vi "EnFlo_Tun_Heater_Control.vi"(1 "Ch Names":string[](array[string]), 2 "Values":dbl[](array[numeric]) format="%.2f") -> ()   [LabVIEW 2010]
uses:
  ADAM_Global.vi
  <vilib>/Analysis/NI_AALPro.lvlib
  <vilib>/Analysis/NI_AALBase.lvlib
panel:
  in  "Total History":i32=80
  out "Proportional Term":dbl format="%#.1f"
  out "Control Sum":dbl format="%#.1f"
  out "Differential Term":dbl format="%#.1f"
  in  "Derivative History":i32=25
  out "Integral Term":dbl format="%#.1f"
  in  "Kp":dbl=6.0 format="%.2f"
  in  "Kd":dbl=150.0 format="%.2f"
  in  "Ki":dbl=0.05 format="%.2f"
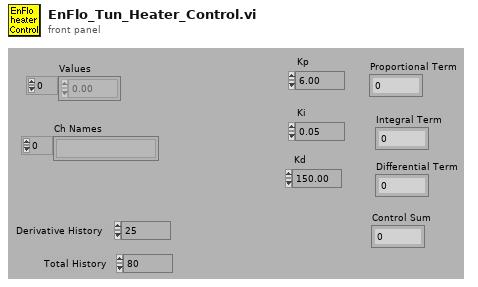
[diagram p1: front panel]
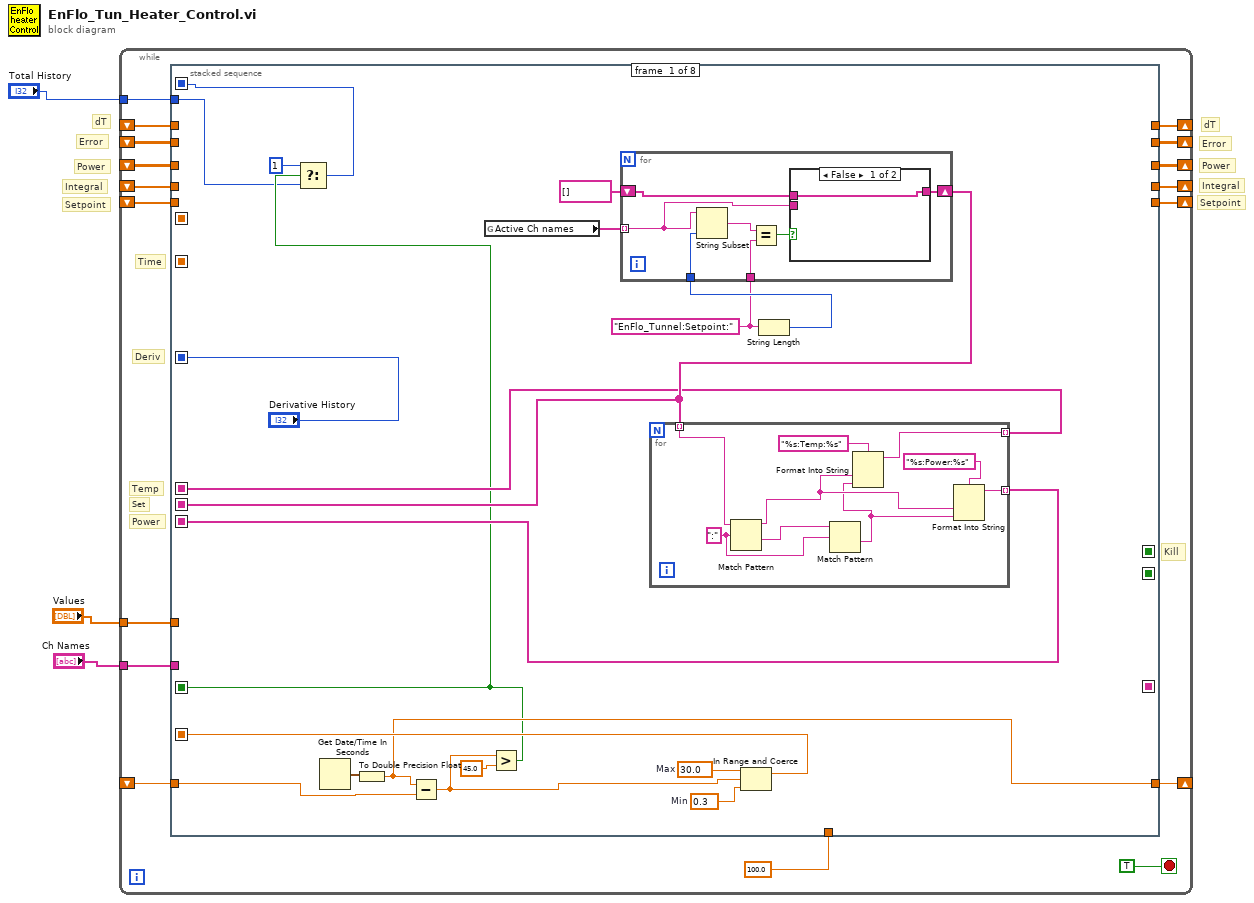
[diagram p0: block diagram]
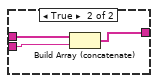
[diagram p2: hidden frame]
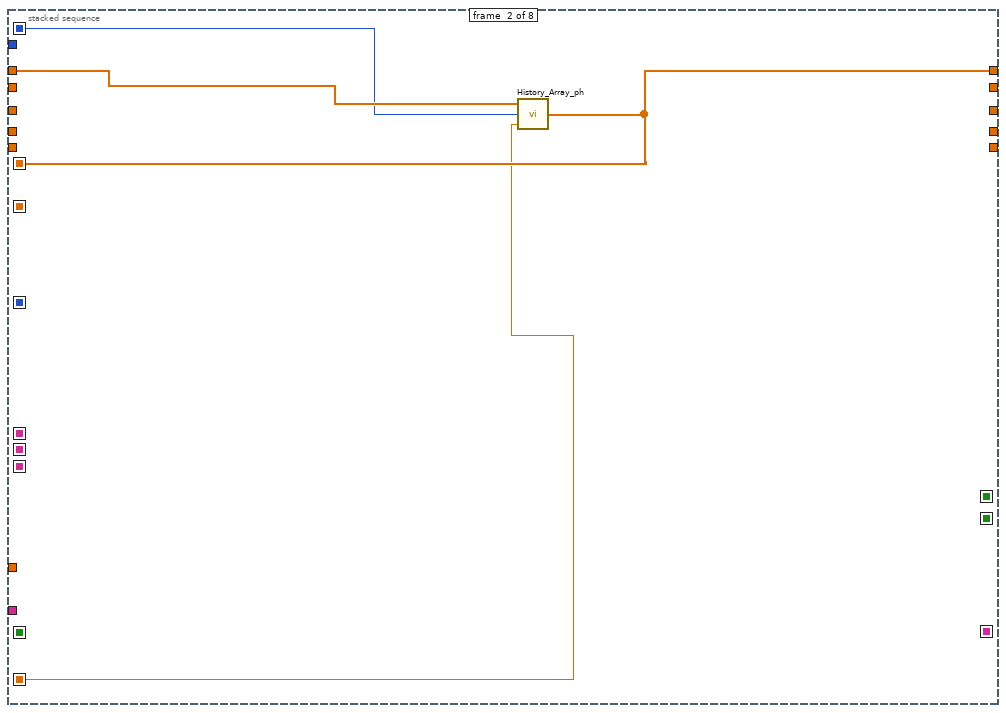
[diagram p3: hidden frame]
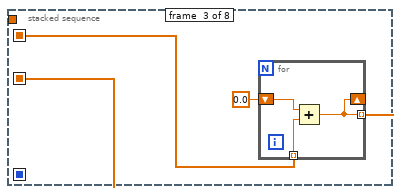
[diagram p4: hidden frame]
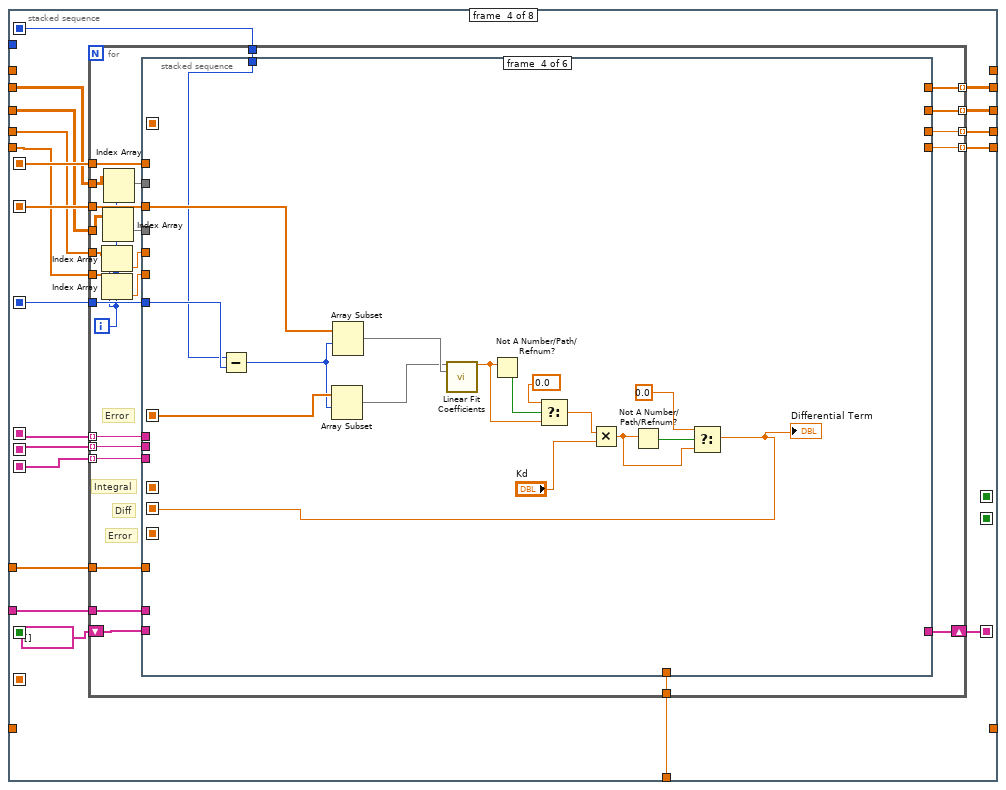
[diagram p5: hidden frame]
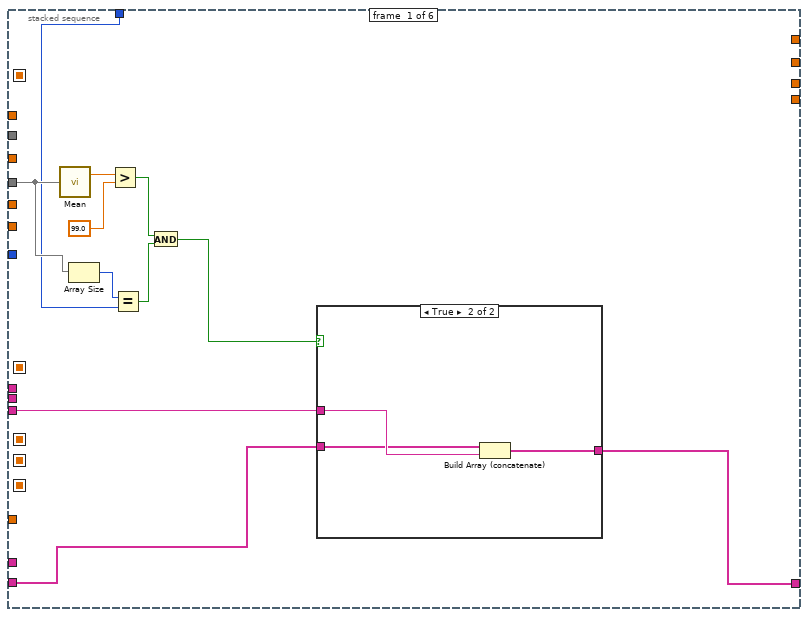
[diagram p6: hidden frame]
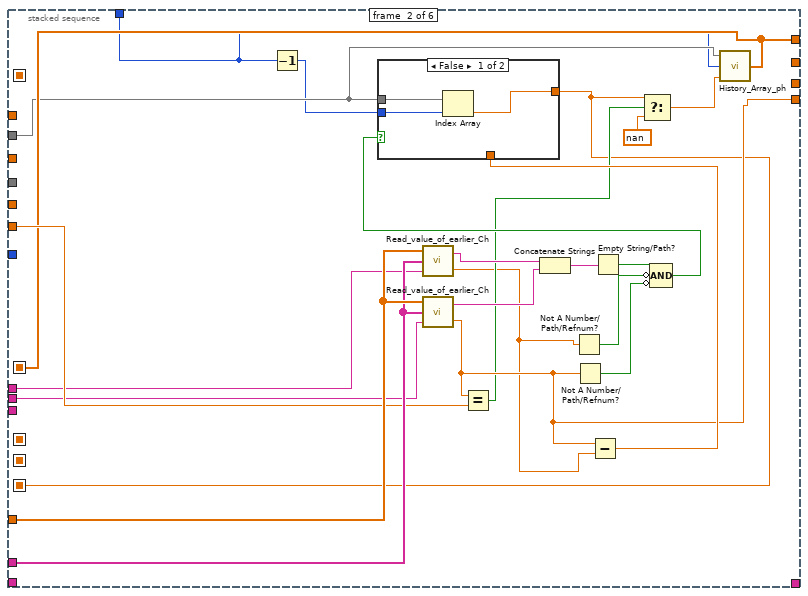
[diagram p8: hidden frame]
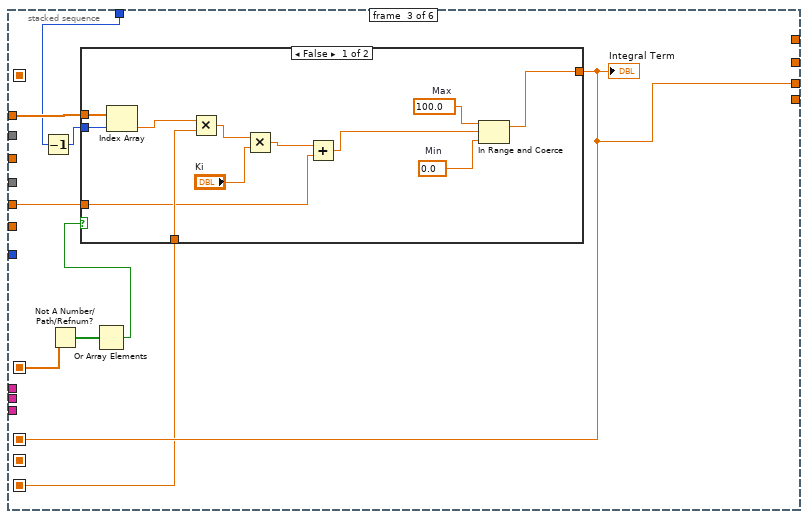
[diagram p10: hidden frame]
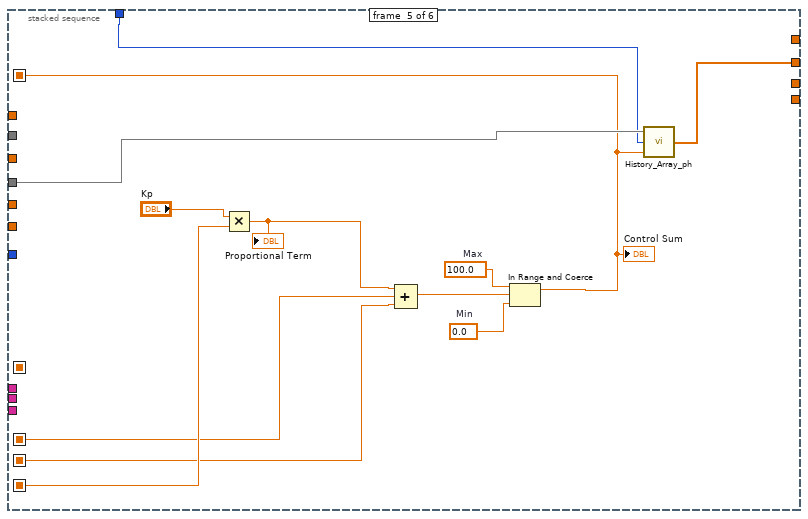
[diagram p12: hidden frame]
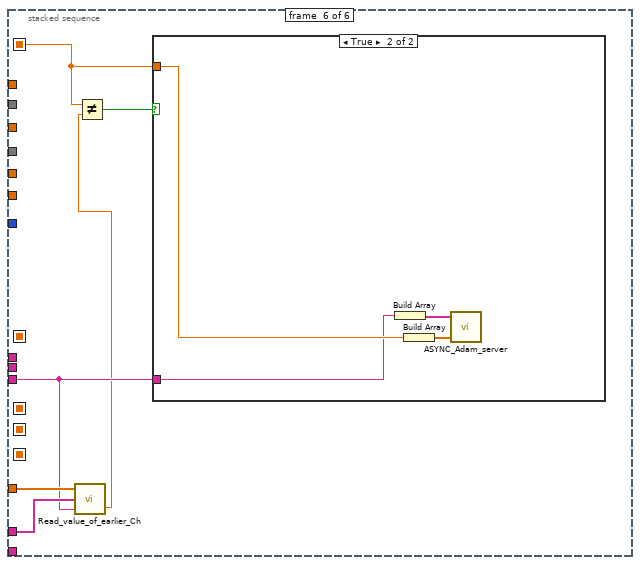
[diagram p13: hidden frame]
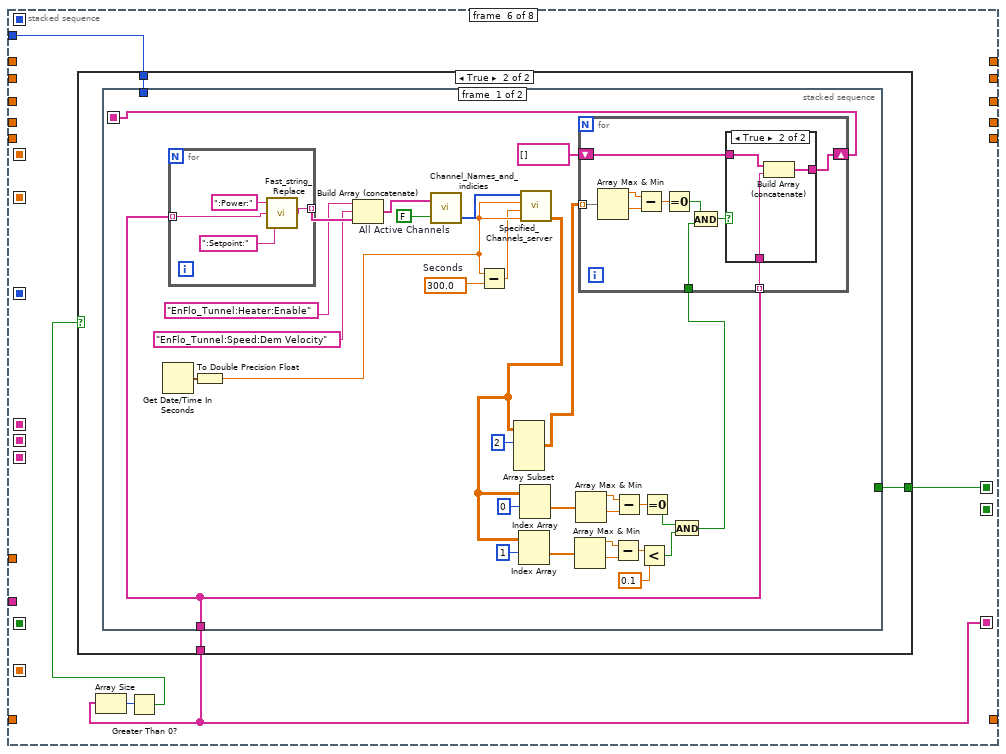
[diagram p16: hidden frame]
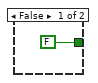
[diagram p17: hidden frame]
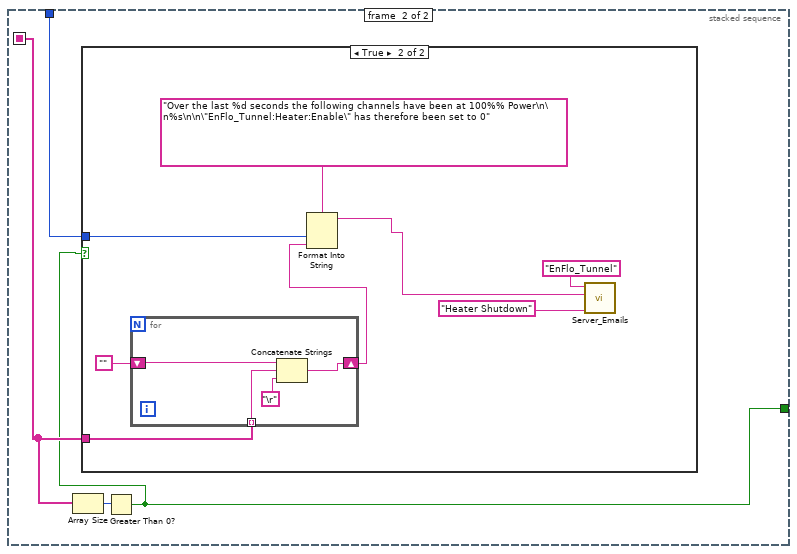
[diagram p19: hidden frame]
diagram:
  # "Setpoint"
  # "Integral"
  # "Power"
  # "Error"
  # "dT"
  # "Setpoint"
  # "Power"
  # "Integral"
  # "Error"
  # "dT"
  n1 = while {
    shift-right: [w18] -> _
    shift-left: _ -> [w19]
    shift-right: [w14] -> _
    shift-left: _ -> [w17]
    shift-right: [w16] -> _
    shift-left: _ -> [w15]
    shift-right: [w12] -> _
    shift-left: _ -> [w13]
    shift-right: [w10] -> _
    shift-left: _ -> [w11]
    shift-right: [w8] -> _
    shift-left: _ -> [w9]
    tunnel: "Total History" -> [w7]
    tunnel: "Ch Names" -> [w5]
    tunnel: "Values" -> [w4]
    stop <- TRUE stop-if-true
    # "Kill"
    # "Power"
    # "Set"
    # "Temp"
    # "Deriv"
    # "Time"
    n2 = stacked-sequence {
      seq-local: [_ w64 _ _ _ _ _ _] -> [_ _ w66 w89 _ _ _ _]
      seq-local: [_ _ w65 _ _ _ _ _] -> [_ _ _ w88 _ _ _ _]
      seq-local: ["Derivative History" _ _ _ _ _ _ _] -> [_ _ _ w84 _ _ _ _]
      seq-local: [w34 _ _ _ _ _ _ _] -> [_ _ _ w83 _ _ _ _]
      seq-local: [w36 _ _ _ _ _ _ _] -> [_ _ _ w82 _ _ _ _]
      seq-local: [w35 _ _ _ _ _ _ _] -> [_ _ _ w81 _ _ _ _]
      seq-local: [_ _ _ w78 _ _ _ _] -> [_ _ _ _ _ w220 _ _]
      seq-local: [_ _ _ _ _ w218 _ _] -> [_ _ _ _ _ _ w299 _]
      seq-local: [_ _ _ _ _ _ w300 _] -> [_ _ _ _ _ _ _ w326]
      seq-local: [w28 _ _ _ _ _ _ _] -> [_ w62 _ _ _ _ _ _]
      seq-local: [w24 _ _ _ _ _ _ _] -> [_ _ _ _ _ _ _ _]
      seq-local: [w22 _ _ _ _ _ _ _] -> [_ w61 _ w71 _ _ _ _]
      tunnel: w19 -> [_ w63 _ _ _ _ _ _]
      tunnel: [_ w64 _ _ _ _ _ _] -> w18
      tunnel: w17 -> [_ _ _ w75 _ _ _ _]
      tunnel: [w25 _ _ _ _ _ _ _] -> w16
      tunnel: w15 -> [w29 _ _ _ _ _ _ _]
      tunnel: [_ _ _ w90 _ _ _ _] -> w14
      tunnel: w13 -> [_ _ _ w74 _ _ _ _]
      tunnel: [_ _ _ w87 _ _ _ _] -> w12
      tunnel: w11 -> [_ _ _ w73 _ _ _ _]
      tunnel: [_ _ _ w86 _ _ _ _] -> w10
      tunnel: w9 -> [_ _ _ w72 _ _ _ _]
      tunnel: [_ _ _ w85 _ _ _ _] -> w8
      tunnel: w7 -> [w23 _ _ _ _ w221 w301 _]
      tunnel: 100.0 ("y") -> [_ _ _ w79 _ _ w293 _]
      tunnel: w5 -> [_ _ _ w77 _ _ w296 _]
      tunnel: w4 -> [_ _ _ w76 _ _ w295 _]
      frame #0 {
        w31 = 0.3  # Min
        w30 = 30.0  # Max
        w38 = "EnFlo_Tunnel:Setpoint:"
        n3 = Get Date/Time In Seconds() -> (seconds since 1Jan1904=w32:timestamp)
        n4 = To Double Precision Float(number=w32) -> (double precision float=w25:dbl)
        n5 = Subtract(x=w25, y=w29) -> (x-y=w27:dbl)
        n6 = global read "ADAM_Global.vi" "Active Ch names"() -> (w40:string[])
        n7 = Greater?(x=w27, y=45.0) -> (0:w24:bool)
        n8 = Select(t=1, s=w24, f=w23) -> (s? t:f=w22:i32)
        n9 = In Range and Coerce(upper limit=w30, x=w27, lower limit=w31) -> (coerced(x)=w28:dbl)  [unwired: 1 out]
        n10 = String Length(string=w38) -> (length=w39:i32)
        n11 = for {
          shift-right: [w41] -> w36
          shift-left: string[] [] -> [w43]
          tunnel: w40 -> [w42] mode=indexing
          tunnel: w39 -> [w47]
          tunnel: w38 -> [w46]
          n12 = String Subset(string=w42, length (rest)=w47) -> (substring=w45:string)  [unwired: 1 out]
          n13 = Equal?(x=w45, y=w46) -> (x = y?=w44:bool)
          n14 = case shown="False" w44 {
            tunnel: w43 -> [w48 w51]
            tunnel: w42 -> [_ w50]
            tunnel: [w48 w49] -> w41
            frame False {
            }
            frame True {
              n15 = Build Array (concatenate)(w51, w50) -> (w49:string[])
            }
          }
        }
        n16 = for {
          tunnel: w36 -> [w52] mode=indexing
          tunnel: [w53] -> w35 mode=indexing
          tunnel: [w54] -> w34 mode=indexing
          w59 = ":" ("regular expression")
          n17 = Match Pattern(string=w52, regular expression=w59) -> (before substring=w56:string, after substring=w60:string)  [unwired: 3 out]
          n18 = Match Pattern(string=w60, regular expression=w59) -> (after substring=w55:string)  [unwired: 4 out]
          n19 = Format Into String(format string="%s:Temp:%s", w56, w55) -> (resulting string=w54:string)  [unwired: 2 in, 1 out]
          n20 = Format Into String(format string="%s:Power:%s", w56, w55) -> (resulting string=w53:string)  [unwired: 2 in, 1 out]
        }
      }
      frame #1 {
        n21 = call "History_Array_ph.vi"("Current Value"=w62, "Desired Length"=w61, "History In"=w63) -> ("History Out"=w64:dbl[])
      }
      frame #2 {
        n22 = for {
          shift-right: [w68] -> _
          shift-left: 0.0 ("element") -> [w70]
          tunnel: w66 -> [w69] mode=indexing
          tunnel: [w68] -> w65 mode=indexing
          n23 = Add(x=w70, y=w69) -> (x+y=w68:dbl)
        }
      }
      frame #3 {
        n24 = for {
          tunnel: w76 -> [w115]
          tunnel: w77 -> [w114]
          tunnel: [w113] -> w90 mode=indexing
          tunnel: w75 -> [w97]
          tunnel: w89 -> [w112]
          tunnel: w88 -> [w99]
          tunnel: [w111] -> w87 mode=indexing
          tunnel: w74 -> [w98]
          tunnel: [w110] -> w86 mode=indexing
          tunnel: w73 -> [w100]
          tunnel: [w109] -> w85 mode=indexing
          tunnel: w72 -> [w94]
          tunnel: w84 -> [w108]
          tunnel: w83 -> [w107] mode=indexing
          tunnel: w82 -> [w106] mode=indexing
          tunnel: w81 -> [w105] mode=indexing
          shift-right: [w103] -> w78
          shift-left: string[] [] -> [w104]
          tunnel: w79 -> [w102]
          tunnel: w71 -> [w91]
          i -> [w92]
          # "Integral"
          # "Error"
          # "Error"
          # "Diff"
          n25 = Index Array(array=w100, index=w92) -> (element=w101:dbl)
          n26 = Index Array(array=w94, index=w92) -> (element=w93:dbl)
          n27 = Index Array(array=w98, index (row)=w92) -> (element=w95:dbl[])  [unwired: 1 in]
          n28 = Index Array(array=w97, index (row)=w92) -> (element=w96:dbl[])  [unwired: 1 in]
          n29 = stacked-sequence {
            seq-local: [_ _ _ w189 _ _] -> [_ _ _ _ w203 _]
            seq-local: [_ w140 _ _ _ _] -> [_ _ w164 _ w207 _]
            seq-local: [_ w135 _ _ _ _] -> [_ _ w162 w184 _ _]
            seq-local: [_ _ w166 _ _ _] -> [_ _ _ _ w204 _]
            seq-local: [_ _ _ _ w197 _] -> [_ _ _ _ _ w212]
            tunnel: w115 -> [_ w153 _ _ _ w211]
            tunnel: w114 -> [_ w152 _ _ _ w210]
            tunnel: [_ w135 _ _ _ _] -> w113
            tunnel: w96 -> [_ w134 _ _ _ _]
            tunnel: w112 -> [_ _ w165 _ _ _]
            tunnel: w99 -> [_ _ _ w186 _ _]
            tunnel: [_ _ _ _ w199 _] -> w111
            tunnel: w95 -> [w124 _ _ _ w198 _]
            tunnel: [_ _ w166 _ _ _] -> w110
            tunnel: w101 -> [_ _ w163 _ _ _]
            tunnel: [_ w143 _ _ _ _] -> w109
            tunnel: w93 -> [_ w142 _ _ _ _]
            tunnel: w108 -> [_ _ _ w181 _ _]
            tunnel: w107 -> [_ w136 _ _ _ _]
            tunnel: w106 -> [_ w138 _ _ _ _]
            tunnel: w105 -> [w119 _ _ _ _ w209]
            tunnel: w104 -> [w118 _ _ _ _ _]
            tunnel: [w117 _ _ _ _ _] -> w103
            tunnel: w102 -> [_ _ _ _ _ _]
            tunnel: w91 -> [w116 w132 w159 w180 w196 _]
            frame #0 {
              n30 = call <vilib>:"Mean.vi"("X"=w124) -> ("mean"=w126:dbl)  [unwired: 1 out]
              n31 = Array Size(array=w124) -> (size(s)=w123:i32)
              n32 = Greater?(x=w126, y=99.0) -> (0:w121:bool)
              n33 = Equal?(x=w123, y=w116) -> (x = y?=w122:bool)
              n34 = And(x=w121, y=w122) -> (x .and. y?=w120:bool)
              n35 = case shown="True" w120 {
                tunnel: w119 -> [_ w130]
                tunnel: w118 -> [w127 w129]
                tunnel: [w127 w128] -> w117
                frame False {
                }
                frame True {
                  n36 = Build Array (concatenate)(w129, w130) -> (w128:string[])
                }
              }
            }
            frame #1 {
              n37 = Decrement(x=w132) -> (x-1=w131:i32)
              n38 = call "Read_value_of_earlier_Ch.vi"("Desired Ch to Read"=w136, "Ch names"=w152, "Present scan array"=w153) -> ("Value"=w137:dbl, "Scan comment"=w151:string)  [unwired: 1 in]
              n39 = call "Read_value_of_earlier_Ch.vi"("Desired Ch to Read"=w138, "Ch names"=w152, "Present scan array"=w153) -> ("Value"=w143:dbl, "Scan comment"=w150:string)  [unwired: 1 in]
              n40 = Equal?(x=w143, y=w142) -> (x = y?=w141:bool)
              n41 = Concatenate Strings(w151, w150) -> (w149:string)
              n42 = Not A Number/Path/Refnum?(number/path/refnum=w137) -> (NaN/Path/Refnum?=w147:bool)
              n43 = Not A Number/Path/Refnum?(number/path/refnum=w143) -> (NaN/Path/Refnum?=w146:bool)
              n44 = Subtract(x=w143, y=w137) -> (x-y=w144:dbl)
              n45 = Empty String/Path?(string/path=w149) -> (empty?=w148:bool)
              n46 = Compound Arithmetic op=AND(w148, invert w147, invert w146) -> (w145:bool)
              n47 = case shown="False" w145 {
                tunnel: w131 -> [w156 _]
                tunnel: w134 -> [w155 _]
                tunnel: [w154 w157] -> w140
                tunnel: w144 -> [_ w157]
                frame False {
                  n48 = Index Array(array=w155, index=w156) -> (element=w154:dbl)
                }
                frame True {
                }
              }
              n49 = Select(t=w140, s=w141, f=nan) -> (s? t:f=w133:dbl)
              n50 = call "History_Array_ph.vi"("Current Value"=w133, "Desired Length"=w132, "History In"=w134) -> ("History Out"=w135:dbl[])
            }
            frame #2 {
              n51 = Decrement(x=w159) -> (x-1=w158:i32)
              n52 = Not A Number/Path/Refnum?(number/path/refnum=w162) -> (NaN/Path/Refnum?=w161:bool[])
              n53 = Or Array Elements(Boolean array=w161) -> (logical OR=w160:bool)
              n54 = case shown="False" w160 {
                tunnel: [w175 w179] -> w166
                tunnel: w158 -> [w174 _]
                tunnel: w165 -> [w173 _]
                tunnel: w164 -> [w171 _]
                tunnel: w163 -> [w169 w179]
                frame False {
                  w178 = 0.0  # Min
                  w176 = 100.0  # Max
                  n55 = Index Array(array=w173, index=w174) -> (element=w172:dbl)
                  n56 = Multiply(x=w172, y=w171) -> (x*y=w170:dbl)
                  n57 = Multiply(x=w170, y="Ki") -> (x*y=w168:dbl)
                  n58 = Add(x=w168, y=w169) -> (x+y=w167:dbl)
                  n59 = In Range and Coerce(upper limit=w176, x=w167, lower limit=w178) -> (coerced(x)=w175:dbl)  [unwired: 1 out]
                }
                frame True {
                }
              }
              "Integral Term" <- w166
            }
            frame #3 {
              n60 = Subtract(x=w180, y=w181) -> (x-y=w182:i32)
              n61 = Array Subset(array=w184, index=w182) -> (w183:dbl[])  [unwired: 1 in]
              n62 = Array Subset(array=w186, index=w182) -> (w185:dbl[])  [unwired: 1 in]
              n63 = call <vilib>:"Linear Fit Coefficients.vi"("Y"=w183, "X"=w185) -> ("slope"=w195:dbl)  [unwired: 3 in, 10 out]
              n64 = Not A Number/Path/Refnum?(number/path/refnum=w195) -> (NaN/Path/Refnum?=w193:bool)
              n65 = Select(t=0.0 ("f"), s=w193, f=w195) -> (s? t:f=w192:dbl)
              n66 = Multiply(x=w192, y="Kd") -> (x*y=w188:dbl)
              n67 = Not A Number/Path/Refnum?(number/path/refnum=w188) -> (NaN/Path/Refnum?=w190:bool)
              n68 = Select(t=0.0, s=w190, f=w188) -> (s? t:f=w189:dbl)
              "Differential Term" <- w189
            }
            frame #4 {
              w202 = 0.0  # Min
              w201 = 100.0  # Max
              n69 = Multiply(x="Kp", y=w207) -> (x*y=w205:dbl)
              "Proportional Term" <- w205
              n70 = Compound Arithmetic op=ADD(w205, w204, w203) -> (w200:dbl)
              n71 = In Range and Coerce(upper limit=w201, x=w200, lower limit=w202) -> (coerced(x)=w197:dbl)  [unwired: 1 out]
              "Control Sum" <- w197
              n72 = call "History_Array_ph.vi"("Current Value"=w197, "Desired Length"=w196, "History In"=w198) -> ("History Out"=w199:dbl[])
            }
            frame #5 {
              n73 = call "Read_value_of_earlier_Ch.vi"("Desired Ch to Read"=w209, "Ch names"=w210, "Present scan array"=w211) -> ("Value"=w208:dbl)  [unwired: 1 in, 1 out]
              n74 = Not Equal?(x=w212, y=w208) -> (x != y?=w213:bool)
              n75 = case shown="True" w213 {
                tunnel: w212 -> [_ w215]
                tunnel: w209 -> [_ w214]
                frame False {
                }
                frame True {
                  n76 = Build Array(w214) -> (w216:string[])
                  n77 = Build Array(w215) -> (w217:dbl[])
                  n78 = call "ASYNC_Adam_server.vi"("Values"=w217, "Channel Names"=w216) -> ()  [unwired: 1 in, 3 out]
                }
              }
            }
          }
        }
      }
      frame #4 {
      }
      frame #5 {
        n79 = Array Size(array=w220) -> (size(s)=w222:i32)
        n80 = Greater Than 0?(x=w222) -> (x > 0?=w219:bool)
        n81 = case shown="True" w219 {
          tunnel: w221 -> [_ w225]
          tunnel: w220 -> [_ w226]
          tunnel: [FALSE w224] -> w218
          frame False {
          }
          frame True {
            n82 = stacked-sequence {
              seq-local: [w251 _] -> [_ w276]
              tunnel: w226 -> [w250 _]
              tunnel: w225 -> [_ w278]
              tunnel: [_ w275] -> w224
              frame #0 {
                w254 = 300.0  # Seconds
                w256 = FALSE  # All Active Channels
                n83 = Get Date/Time In Seconds() -> (seconds since 1Jan1904=w253:timestamp)
                n84 = for {
                  tunnel: w250 -> [w272] mode=indexing
                  tunnel: [w271] -> w247 mode=indexing
                  n85 = call "Fast_string_Replace.vi"("Replace match with:"=":Setpoint:" ("regular expression"), "Input String"=w272, "regular expression"=":Power:") -> ("Output String"=w271:string)  [unwired: 2 out]
                }
                n86 = To Double Precision Float(number=w253) -> (double precision float=w249:dbl)
                n87 = Build Array (concatenate)("EnFlo_Tunnel:Heater:Enable", "EnFlo_Tunnel:Speed:Dem Velocity", w247) -> (w245:string[])
                n88 = call "Channel_Names_and_indicies.vi"("All Active Channels"=w256, "Desired Ch Names"=w245) -> ("Indicies"=w255:i32[])  [unwired: 1 out]
                n89 = Subtract(x=w249, y=w254) -> (x-y=w248:dbl)
                n90 = call "Specified_Channels_server.vi"("End time"=w249, "Start time"=w248, "Clients time"=w249, "Requested channels"=w255) -> ("Output array"=w232:dbl[][])  [unwired: 1 in, 4 out]
                n91 = Array Subset(array=w232, index (row)=2 ("index")) -> (w243:dbl[][])  [unwired: 3 in]
                n92 = Index Array(array=w232, index (row)=1) -> (element=w237:dbl[])  [unwired: 1 in]
                n93 = Index Array(array=w232, index (row)=0) -> (element=w239:dbl[])  [unwired: 1 in]
                n94 = Array Max & Min(array=w237) -> (max value=w235:dbl, min value=w236:dbl)  [unwired: 2 out]
                n95 = Array Max & Min(array=w239) -> (max value=w241:dbl, min value=w240:dbl)  [unwired: 2 out]
                n96 = Subtract(x=w235, y=w236) -> (x-y=w229:dbl)
                n97 = Subtract(x=w241, y=w240) -> (x-y=w242:dbl)
                n98 = Less?(x=w229, y=0.1) -> (x < y?=w227:bool)
                n99 = Equal To 0?(x=w242) -> (x = 0?=w231:bool)
                n100 = And(x=w231, y=w227) -> (x .and. y?=w230:bool)
                n101 = for {
                  tunnel: w243 -> [w266] mode=indexing
                  shift-right: [w260] -> w251
                  shift-left: string[] [] -> [w261]
                  tunnel: w250 -> [w262] mode=indexing
                  tunnel: w230 -> [w257]
                  n102 = Array Max & Min(array=w266) -> (max value=w264:dbl, min value=w265:dbl)  [unwired: 2 out]
                  n103 = Subtract(x=w264, y=w265) -> (x-y=w263:dbl)
                  n104 = Equal To 0?(x=w263) -> (x = 0?=w259:bool)
                  n105 = And(x=w259, y=w257) -> (x .and. y?=w258:bool)
                  n106 = case shown="True" w258 {
                    tunnel: w262 -> [_ w270]
                    tunnel: w261 -> [w267 w269]
                    tunnel: [w267 w268] -> w260
                    frame False {
                    }
                    frame True {
                      n107 = Build Array (concatenate)(w269, w270) -> (w268:string[])
                    }
                  }
                }
              }
              frame #1 {
                n108 = Array Size(array=w276) -> (size(s)=w277:i32)
                n109 = Greater Than 0?(x=w277) -> (x > 0?=w275:bool)
                n110 = case shown="True" w275 {
                  tunnel: w278 -> [_ w282]
                  tunnel: w276 -> [_ w279]
                  frame False {
                  }
                  frame True {
                    n111 = for {
                      shift-right: [w287] -> w283
                      shift-left: "" -> [w290]
                      tunnel: w279 -> [w288] mode=indexing
                      n112 = Concatenate Strings(w290, w288, "\r") -> (w287:string)
                    }
                    n113 = Format Into String(format string="Over the last %d seconds the following channels have been at 100%% Power\n\n%s\n\n\"EnFlo_Tunnel:Heater:Enable\" has therefore been set to 0", w282, w283) -> (resulting string=w280:string)  [unwired: 2 in, 1 out]
                    n114 = call "Server_Emails.vi"("Client Name Contains"="EnFlo_Tunnel", "Message"=w280, "Subject"="Heater Shutdown" ("t")) -> ()  [unwired: 2 in, 3 out]
                  }
                }
              }
            }
          }
        }
      }
      frame #6 {
        w297 = "EnFlo_Tunnel:Temp:"
        n115 = String Length(string=w297) -> (length=w298:i32)
        n116 = for {
          shift-right: [w307] -> w291
          shift-left: "" -> [w308]
          tunnel: w296 -> [w311] mode=indexing
          tunnel: w298 -> [w312]
          tunnel: w297 -> [w309]
          tunnel: w295 -> [w306] mode=indexing
          tunnel: w293 -> [w305]
          n117 = String Subset(string=w311, length (rest)=w312) -> (substring=w310:string)  [unwired: 1 out]
          n118 = Equal?(x=w310, y=w309) -> (x = y?=w302:bool)
          n119 = Greater?(x=w306, y=w305) -> (0:w303:bool)
          n120 = And(x=w302, y=w303) -> (x .and. y?=w304:bool)
          n121 = case shown="False" w304 {
            tunnel: w311 -> [_ w314]
            tunnel: w308 -> [w313 w316]
            tunnel: [w313 w315] -> w307
            frame False {
            }
            frame True {
              n122 = Concatenate Strings(w316, w314, "\r") -> (w315:string)
            }
          }
        }
        n123 = Empty String/Path?(string/path=w291) -> (empty?=w292:bool)
        n124 = case shown="False" w292 {
          tunnel: w301 -> [_ _]
          tunnel: w293 -> [w319 _]
          tunnel: [TRUE w325] -> w300
          tunnel: w299 -> [_ w325]
          tunnel: w291 -> [w318 _]
          frame False {
            n125 = Format Into String(format string="The following channels have reached a temperature of  %d deg C\n\n%s\n\n\"EnFlo_Tunnel:Heater:Enable\" has therefore been set to 0", w319, w318) -> (resulting string=w321:string)  [unwired: 2 in, 1 out]
            n126 = call "Server_Emails.vi"("Client Name Contains"="EnFlo_Tunnel", "Message"=w321, "Subject"="Heater Shutdown" ("t")) -> ()  [unwired: 2 in, 3 out]
          }
          frame True {
          }
        }
      }
      frame #7 {
        n127 = case shown="True" w326 {
          frame False {
          }
          frame True {
            n128 = Build Array("EnFlo_Tunnel:Heater:Enable") -> (w329:string[])
            n129 = Build Array(0.0) -> (w327:dbl[])
            n130 = call "ASYNC_Adam_server.vi"("Values"=w327, "Channel Names"=w329) -> ()  [unwired: 1 in, 3 out]
          }
        }
      }
    }
  }
